vi "AWG_UpdateWaveformAndOutput.vi"(8 "Error In":errorcluster, 9 "AWG Sequence":string="const pulse_zeros_head_samples = 1000;\nconst pulse_zeros_tail_samples = 1;\nconst pulse_ones_samples = 500000;\n\nwave wave_pulse_zeros_head = zeros(pulse_zeros_head_samples);\nwave wave_pulse_zeros_tail = zeros(pulse_zeros_tail_samples);\nwave wave_pulse_ones = ones(pulse_ones_samples);\n\nwave wave_pulse = join(wave_pulse_zeros_head, wave_pulse_ones, wave_pulse_zeros_tail);\n\nwhile (true){\n  waitDigTrigger(1);\n  setTrigger(0b1111);\n  playWave(wave_pulse);\n  waitWave();\n  setTrigger(0b0000);\n}", 10 "Selected Device":string, 11 "AWG Handle In":T1 {"Handle" format="0x%08x"; "Conn" format="0x%08x"}) -> (0 "error out":errorcluster, 3 "AWG Handle Out":T1 {"Handle" format="0x%08x"; "Conn" format="0x%08x"})   [LabVIEW 2016, in "ZI AWG.lvlib"]
uses:
  ZI AWG.lvlib
  <instrlib>/Zurich Instruments LabOne/Public/ziTypeHandle.ctl
  <instrlib>/Zurich Instruments LabOne/Public/Modules/ziTypeModEnum.ctl
  <instrlib>/Zurich Instruments LabOne/Public/Modules/ziModSetValueBinary.vi
  <instrlib>/Zurich Instruments LabOne/Public/Configure/ziSetValueDouble.vi
  <instrlib>/Zurich Instruments LabOne/Zurich Instruments LabOne.lvlib
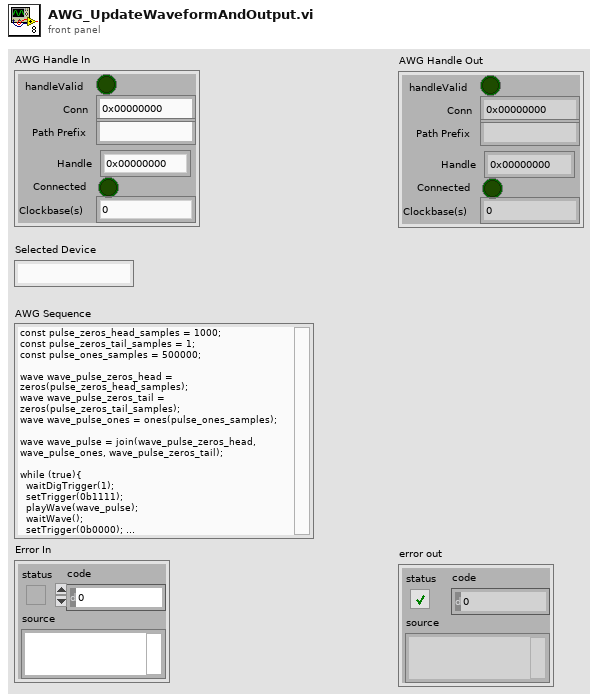
[diagram p1: front panel]
types:
  T1 = typedef "Zurich Instruments LabOne.lvlib/ziTypeHandle.ctl" = cluster{"handleValid":bool, "Conn":u64, "Path Prefix":string, "Handle":u64, "Connected":bool, "Clockbase(s)":dbl}
  T2 = typedef "Zurich Instruments LabOne.lvlib/ziTypeModEnum.ctl" = u16
  T3 = typedef "Zurich Instruments LabOne.lvlib/ziTypeModHandle.ctl" = cluster{"handleValid":bool, "Conn":u64, "ModHandle":u64, "moduleID":string, "Path Prefix":string}
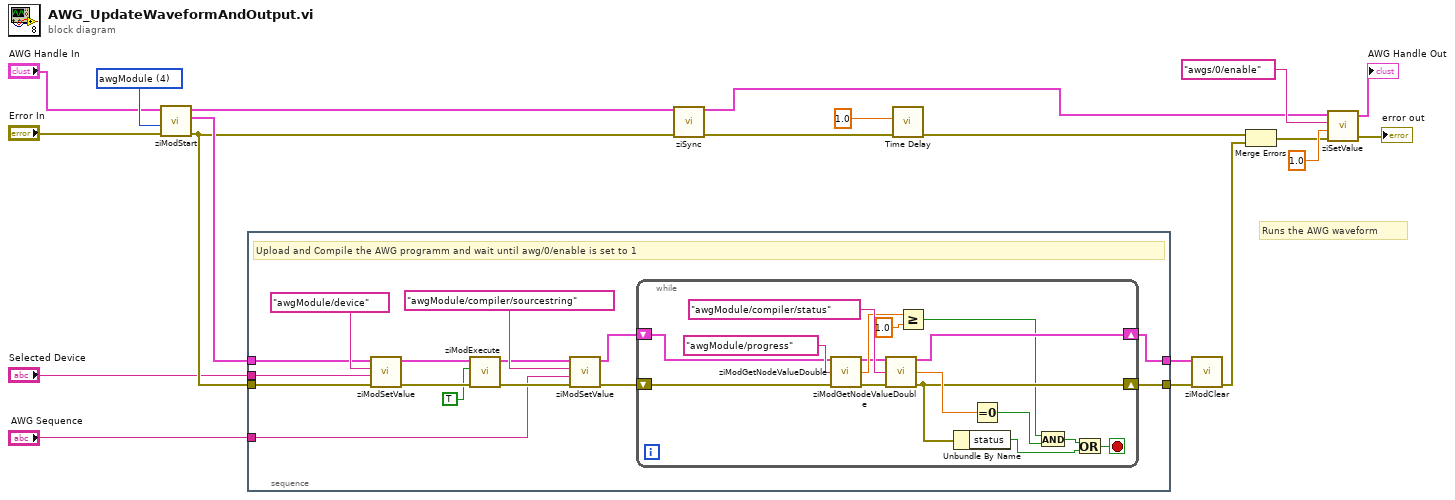
[diagram p0: block diagram]
diagram:
  w15 = T2 4 items=["sweep", "scopeModule", "dataAcquisitionModule", "pidAdvisor", "awgModule", "impedanceModule", "multiDeviceSyncModule", "zoomFFT", "trigger", "deviceSettings", "record"] ("module Id")
  # "Runs the AWG waveform"
  n1 = call <instrlib>:"ziModStart.vi"("Error In"="Error In", "module Id"=w15, "Handle In"="AWG Handle In") -> ("Error Out"=w14:errorcluster, "ModHandle Out"=w18:T3, "Handle Out"=w13:T1)  [unwired: 6 in]
  n2 = stacked-sequence {
    tunnel: [w31] -> w19
    tunnel: [w30] -> w20
    tunnel: w18 -> [w29]
    tunnel: w14 -> [w28]
    tunnel: "Selected Device" -> [w27]
    tunnel: "AWG Sequence" -> [w21]
    frame #0 {
      # "Upload and Compile the AWG programm and wait until awg/0/enable is set to 1"
      n3 = call-poly <instrlib>:"ziModSetValue.vi"("Error In"=w28, "Data"=w27, "Path"="awgModule/device", "ModHandle In"=w29) -> ("Error Out"=w35:errorcluster, "ModHandle Out"=w34:T3)  [unwired: 6 in]
      n4 = call <instrlib>:"ziModExecute.vi"("Error In"=w35, "Modal (F)"=TRUE, "ziModHandle In"=w34) -> ("Error Out"=w24:errorcluster, "ziModHandle Out"=w25:T3)  [unwired: 5 in, 1 out]
      n5 = call-poly <instrlib>:"ziModSetValue.vi"("Error In"=w24, "Data"=w21, "Path"="awgModule/compiler/sourcestring", "ModHandle In"=w25) -> ("Error Out"=w22:errorcluster, "ModHandle Out"=w23:T3)  [unwired: 6 in]
      n6 = while {
        shift-right: [w44] -> w30
        shift-left: w23 -> [w46]
        shift-right: [w39] -> w31
        shift-left: w22 -> [w40]
        stop <- w36 stop-if-true
        n7 = call <instrlib>:"ziModGetNodeValueDouble.vi"("ModHandle In"=w46, "Path"="awgModule/progress", "error in"=w40) -> ("ModHandle Out"=w45:T3, "Value"=w48:dbl, "error out"=w43:errorcluster)  [unwired: 10 in]
        n8 = call <instrlib>:"ziModGetNodeValueDouble.vi"("ModHandle In"=w45, "Path"="awgModule/compiler/status", "error in"=w43) -> ("ModHandle Out"=w44:T3, "Value"=w47:dbl, "error out"=w39:errorcluster)  [unwired: 10 in]
        n9 = Greater Or Equal?(x=w48, y=1.0) -> (x >= y?=w38:bool)
        n10 = Unbundle By Name(w39) -> ("status"=w41:bool)
        n11 = Equal To 0?(x=w47) -> (x = 0?=w37:bool)
        n12 = And(x=w38, y=w37) -> (x .and. y?=w42:bool)
        n13 = Or(x=w42, y=w41) -> (x .or. y?=w36:bool)
      }
    }
  }
  n14 = call <instrlib>:"ziSync.vi"("Handle In"=w13, "Error In"=w14) -> ("Handle Out"=w2:T1, "Error Out"=w11:errorcluster)  [unwired: 12 in]
  n15 = call "Time Delay"("error in (no error)"=w11, "Delay Time (s)"=1.0) -> ("error out"=w9:errorcluster)  [unwired: 9 in]
  n16 = call <instrlib>:"ziModClear.vi"("Error In"=w19, "ziModHandle In"=w20) -> ("Error Out"=w12:errorcluster)  [unwired: 7 in, 1 out]
  n17 = Merge Errors(w9, w12) -> (w10:errorcluster)
  n18 = call-poly <instrlib>:"ziSetValue.vi"("Error In"=w10, "Value"=1.0, "Path"="awgs/0/enable", "Handle In"=w2) -> ("Error Out"=→"error out":errorcluster, "Handle Out"=→"AWG Handle Out":T1)  [unwired: 1 in]
